vi "Write Log Column Header.vi"(8 "error in (no error)":errorcluster, 11 "Model in":refnum<class "Model.lvclass">) -> (0 "error out":errorcluster, 3 "Model out":refnum<class "Model.lvclass">)   [LabVIEW 2016, in "Model.lvclass"]
uses:
  Model.lvclass
  Model.lvclass/Model.ctl
  Test Log/Test Log/OperationsLog.lvclass
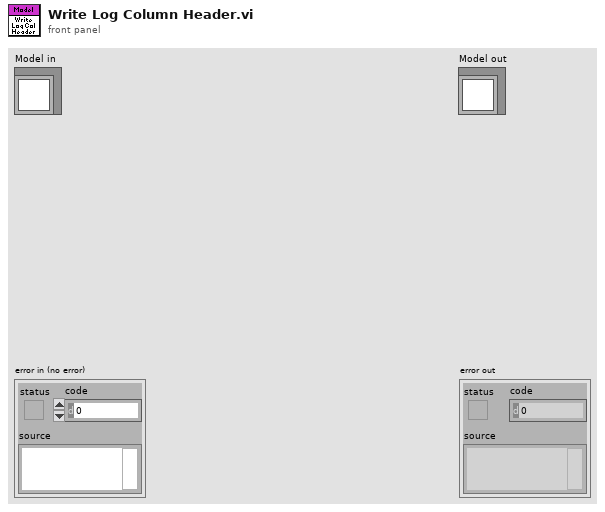
[diagram p1: front panel]
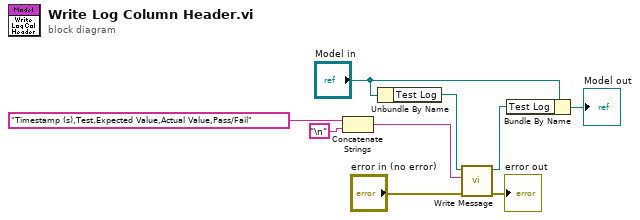
[diagram p0: block diagram]
diagram:
  n1 = Concatenate Strings("Timestamp (s),Test,Expected Value,Actual Value,Pass/Fail" ("format string"), "\n") -> (w2:string)
  n2 = Unbundle By Name("Model in") -> ("Test Log"=w4:refnum<class "OperationsLog.lvclass">)
  n3 = call-dynamic "Write Message.vi"("error in (no error)"="error in (no error)", "Message"=w2, "Test Log in"=w4) -> ("error out"=→"error out":errorcluster, "Test Log out"=w6:refnum<class "OperationsLog.lvclass">)  [unwired: 7 in]
  n4 = Bundle By Name(cluster="Model in", "Test Log"=w6) -> (→"Model out":refnum<class "Model.lvclass">)
